vi "Get Array Element Offsets.vi"(8 "error in (no error)":errorcluster, 9 "Max Index":i32=2147483647, 10 "Offset":i32, 11 "JSON":string="[1,2,3]") -> (0 "error out":errorcluster, 1 "Elements":T1[](array[typedef]), 2 "Offset past Array":i32)   [LabVIEW 2017, in "JSONtext.lvlib"]
uses:
  JSONtext.lvlib
  Parsing/Found Items.ctl
  Parsing/Parsing State.ctl
  Parsing/Advance past String.vi
  Parsing/Advance past Number.vi
  Parsing/Advance past Object.vi
  Parsing/Advance past Array.vi
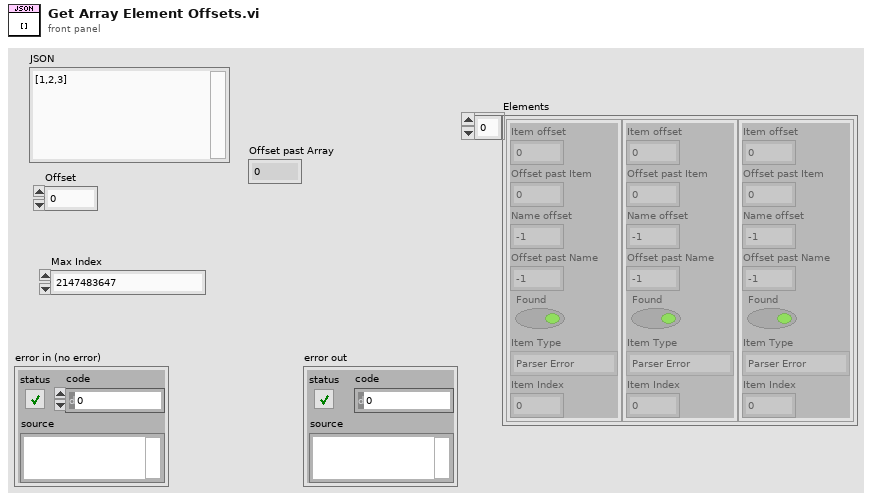
[diagram p1: front panel]
types:
  T1 = typedef "JSONtext.lvlib/Found Items.ctl" = cluster{"Item offset":i32, "Offset past Item":i32, "Name offset":i32, "Offset past Name":i32, "Found":bool, "Item Type":T2, "Item Index":i32}
  T2 = typedef "JSONtext.lvlib/Parsing State.ctl" = enum16{"Parser Error", "Object", "Array", "String", "Number/Other", "Leading Whitespace", "Object end", "Array end", "Value end"}
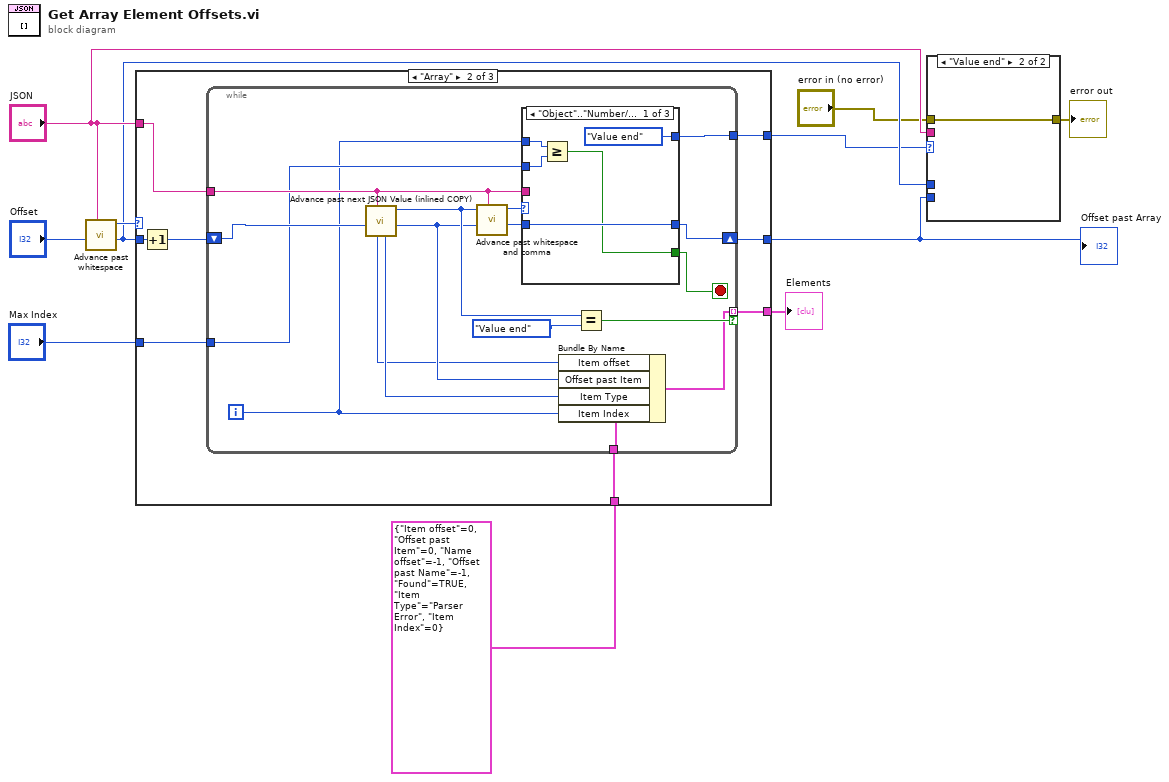
[diagram p0: block diagram]
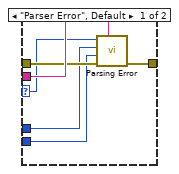
[diagram p2: hidden frame]
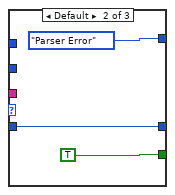
[diagram p4: hidden frame]
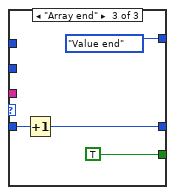
[diagram p5: hidden frame]
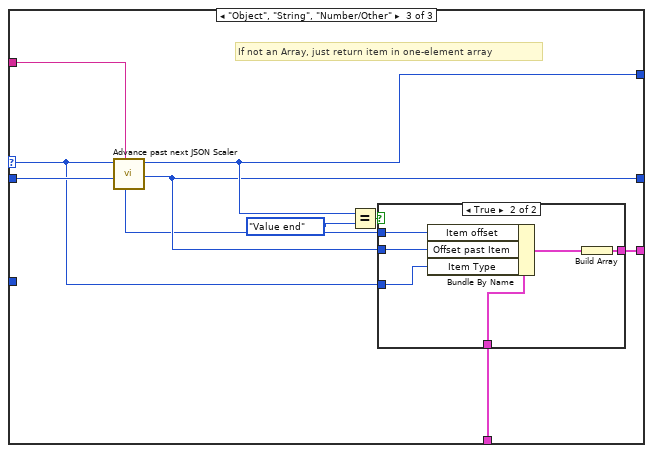
[diagram p6: hidden frame]
diagram:
  n1 = call "Advance past whitespace.vi"("JSON"="JSON", "Offset"="Offset") -> ("Offset of first non-whitespace"=w8:i32, "Parser State"=w10:T2)  [unwired: 8 in]
  n2 = case shown="\"Array\"" w10 {
    selector: w10 -> [w13 _ w53]
    tunnel: [w13 w21 w57] -> w4
    tunnel: [w12 w20 w52] -> w7
    tunnel: [_ w18 w55] -> w3
    tunnel: "JSON" -> [_ w17 w58]
    tunnel: w8 -> [w12 w16 w60]
    tunnel: "Max Index" -> [_ w15 _]
    tunnel: T1 {"Item offset"=0, "Offset past Item"=0, "Name offset"=-1, "Offset past Name"=-1, "Found"=TRUE, "Item Type"=enum."Parser Error", "Item Index"=0} -> [_ w14 w54]
    frame "Parser Error", Default {
    }
    frame "Array" {
      n3 = Increment(x=w16) -> (x+1=w19:i32)
      n4 = while {
        tunnel: w17 -> [w32]
        shift-right: [w35] -> w20
        shift-left: w19 -> [w36]
        tunnel: [w33] -> w21
        tunnel: [w22] -> w18 mode=indexing if=w29
        tunnel: w15 -> [w28]
        tunnel: w14 -> [w27]
        i -> [w26]
        stop <- w34 stop-if-true
        n5 = call "Advance past next JSON Value (inlined COPY).vi"("JSON"=w32, "Offset"=w36) -> ("Offset"=w24:i32, "State"=w30:T2, "Type"=w25:T2, "Value start"=w23:i32)  [unwired: 5 in, 1 out]
        n6 = call "Advance past whitespace and comma.vi"("JSON"=w32, "Offset"=w24, "State in"=w30) -> ("Offset past match"=w38:i32, "State"=w37:T2)  [unwired: 7 in]
        n7 = case shown="\"Object\"..\"Number/Other\"" w37 {
          tunnel: [w40 TRUE TRUE] -> w34
          tunnel: [Parsing_State."Value end" Parsing_State."Parser Error" Parsing_State."Value end"] -> w33
          tunnel: w38 -> [w43 w44 w48]
          tunnel: [w43 w44 w47] -> w35
          tunnel: w32 -> [_ _ _]
          tunnel: w26 -> [w41 _ _]
          tunnel: w28 -> [w42 _ _]
          frame "Object".."Number/Other" {
            n8 = Greater Or Equal?(x=w41, y=w42) -> (x >= y?=w40:bool)
          }
          frame Default {
          }
          frame "Array end" {
            n9 = Increment(x=w48) -> (x+1=w47:i32)
          }
        }
        n10 = Bundle By Name(cluster=w27, "Item offset"=w23, "Offset past Item"=w24, "Item Type"=w25, "Item Index"=w26) -> (w22:T1)
        n11 = Equal?(x=w30, y=Parsing_State."Value end") -> (x = y?=w29:bool)
      }
    }
    frame "Object", "String", "Number/Other" {
      # "If not an Array, just return item in one-element array"
      n12 = call "Advance past next JSON Scaler.vi"("JSON"=w58, "Offset"=w60, "Parser State in"=w53) -> ("Offset Past"=w52:i32, "Parser State"=w57:T2, "Value start"=w51:i32)  [unwired: 6 in]
      n13 = Equal?(x=w57, y=Parsing_State."Value end") -> (x = y?=w56:bool)
      n14 = case shown="True" w56 {
        tunnel: [_ w66] -> w55
        tunnel: w54 -> [_ w65]
        tunnel: w53 -> [_ w64]
        tunnel: w52 -> [_ w63]
        tunnel: w51 -> [_ w62]
        frame False {
        }
        frame True {
          n15 = Bundle By Name(cluster=w65, "Item offset"=w62, "Offset past Item"=w63, "Item Type"=w64) -> (w61:T1)
          n16 = Build Array(w61) -> (w66:T1[])
        }
      }
    }
  }
  "Offset past Array" <- w7
  "Elements" <- w3
  n17 = case shown="\"Value end\"" w4 {
    selector: w4 -> [w67 _]
    tunnel: "JSON" -> [w72 _]
    tunnel: "error in (no error)" -> [w71 w73]
    tunnel: [w70 w73] -> w6
    tunnel: w8 -> [w69 _]
    tunnel: w7 -> [w68 _]
    frame "Parser Error", Default {
      n18 = call "Parsing Error.vi"("JSON"=w72, "error in (no error)"=w71, "Offset past match"=w68, "Value start"=w69, "State"=w67) -> ("error out"=w70:errorcluster)  [unwired: 6 in]
    }
    frame "Value end" {
    }
  }
  "error out" <- w6
